vi "http handle content data.vi"(6 "exec queue":refnum<queue>, 9 "server properties":T1={"max url size"=8000, "max header"=8000, "timeout ms"=5000, "max data size"=104857600}, 10 "application request":T2, 11 "TCP Network Connection in":refnum<k5>) -> (3 "abort":bool)   [LabVIEW 2016, in "Basic HTTP server.lvclass"]
uses:
  Basic HTTP server.lvclass
  http request.ctl
  http method.ctl
  HTTP headers/http header data.ctl
  http server properties.ctl
  http chunked encoding state.ctl
  <vilib>/dlg_ctls.llb/Space Constant.vi
  HTTP headers/http add header to set.vi
  HTTP headers/http headers.lvlib
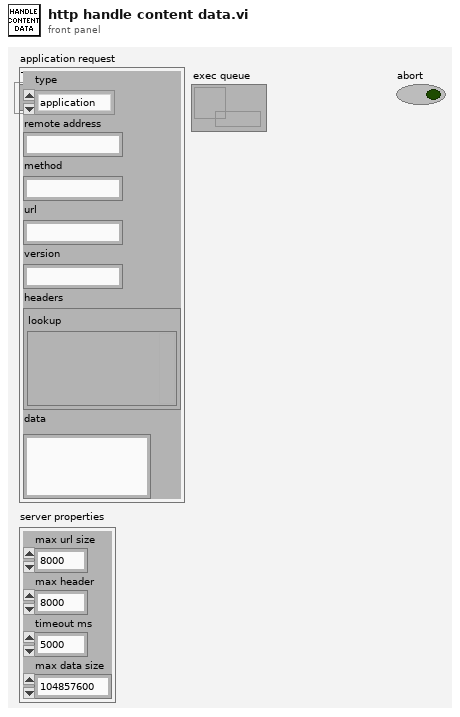
[diagram p1: front panel]
types:
  T1 = typedef "Basic HTTP server.lvclass/http server properties.ctl" = cluster{"max url size":i32, "max header":i32, "timeout ms":i32, "max data size":i32}
  T2 = typedef "Basic HTTP server.lvclass/http request.ctl" = cluster{"type":T3, "remote address":string, "method":string, "url":string, "version":string, "headers":T4, "data":string}
  T3 = typedef "Basic HTTP server.lvclass/http method.ctl" = enum16{"application", "error", "upgrade", "expect"}
  T4 = typedef "http headers.lvlib/http header data.ctl" = cluster{"lookup":variant}
  T5 = typedef "Basic HTTP server.lvclass/http chunked encoding state.ctl" = enum16{"length", "data", "trailer"}
  T6 = enum16{"Standard", "Buffered", "CRLF", "Immediate"}
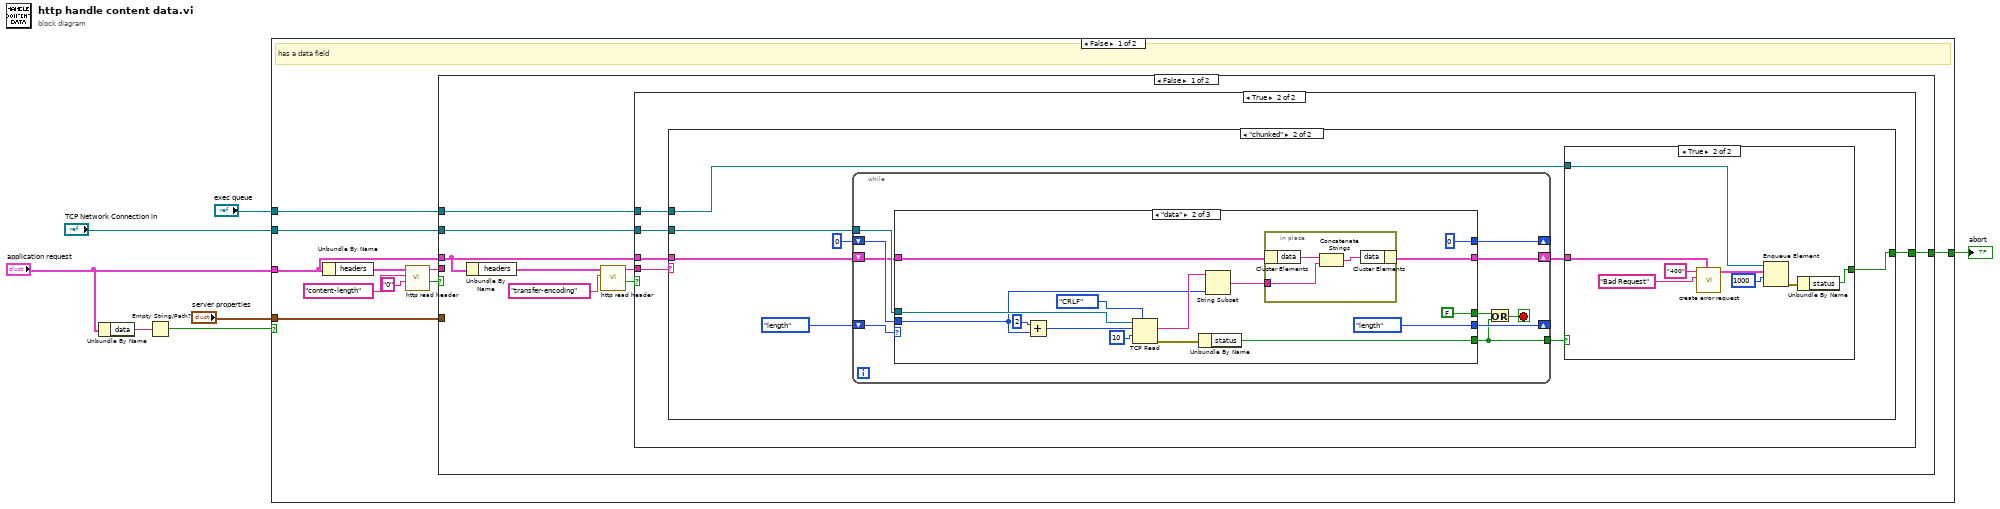
[diagram p0: block diagram]
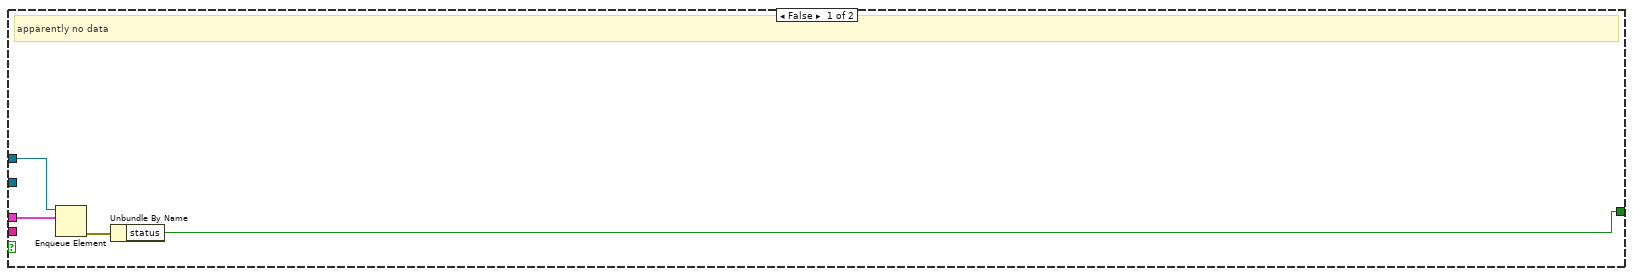
[diagram p2: hidden frame]
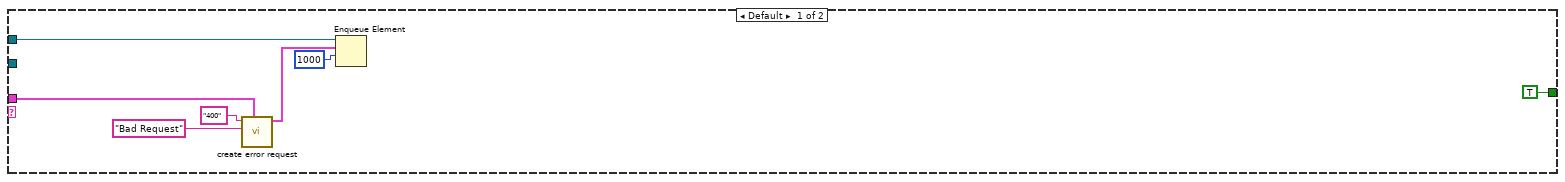
[diagram p3: hidden frame]
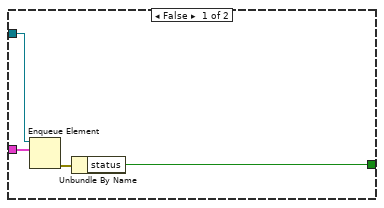
[diagram p4: hidden frame]
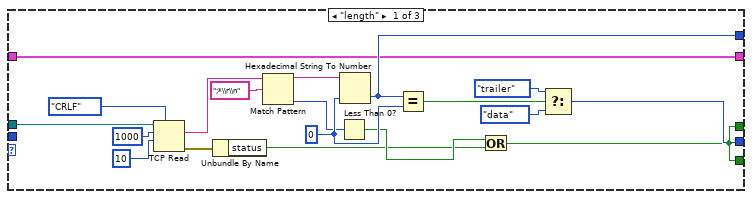
[diagram p5: hidden frame]
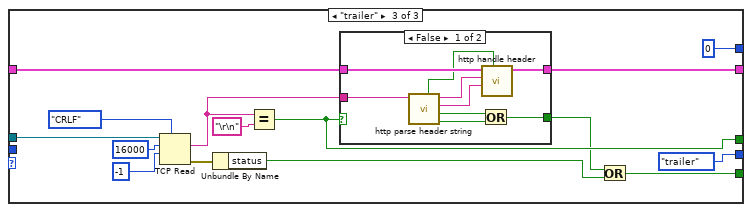
[diagram p6: hidden frame]
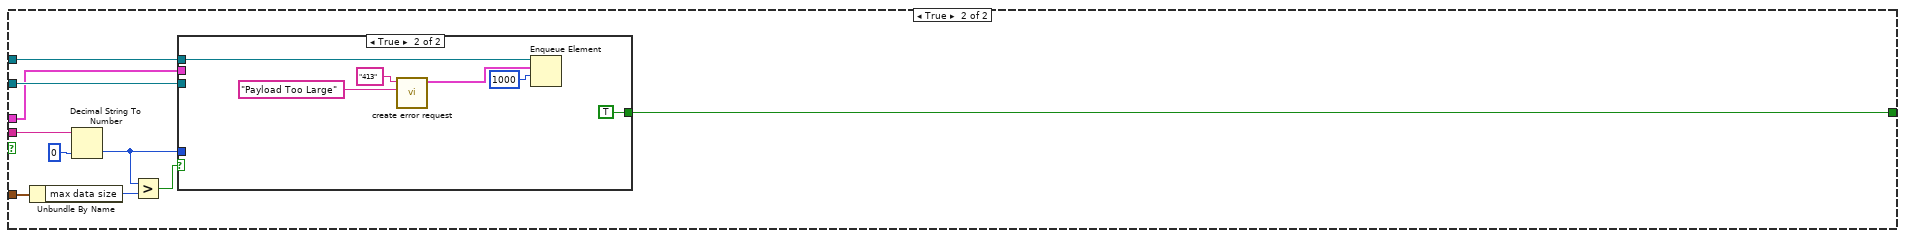
[diagram p8: hidden frame]
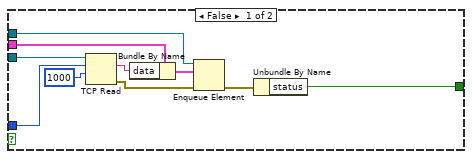
[diagram p9: hidden frame]
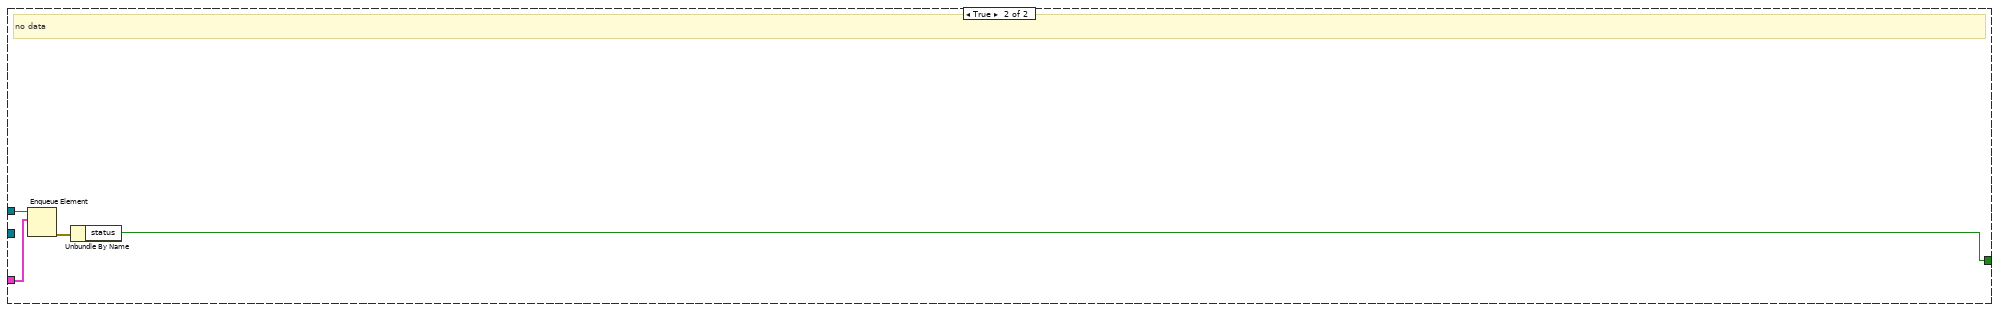
[diagram p10: hidden frame]
diagram:
  n1 = Unbundle By Name("application request") -> ("data"=w2:string)
  n2 = Empty String/Path?(string/path=w2) -> (empty?=w1:bool)
  n3 = case shown="False" w1 {
    tunnel: "TCP Network Connection in" -> [w17 _]
    tunnel: [w16 w160] -> w6
    tunnel: "server properties" -> [w15 _]
    tunnel: "exec queue" -> [w14 w162]
    tunnel: "application request" -> [w13 w163]
    frame False {
      # "has a data field"
      n4 = Unbundle By Name(w13) -> ("headers"=w12:T4)
      n5 = call "http read header.vi"("default value"="0", "header field name"="content-length" ("name"), "headers"=w12) -> ("found"=w10:bool, "value"=w9:string)  [unwired: 7 in]
      n6 = case shown="False" w10 {
        tunnel: w13 -> [w24 w135]
        tunnel: w17 -> [w23 w142]
        tunnel: [w25 w141] -> w16
        tunnel: w15 -> [_ w140]
        tunnel: w14 -> [w22 w136]
        tunnel: w9 -> [_ w134]
        frame False {
          n7 = Unbundle By Name(w24) -> ("headers"=w21:T4)
          n8 = call "http read header.vi"("header field name"="transfer-encoding" ("name"), "headers"=w21) -> ("found"=w19:bool, "value"=w18:string)  [unwired: 8 in]
          n9 = case shown="True" w19 {
            tunnel: [w26 w34] -> w25
            tunnel: w24 -> [w29 w31]
            tunnel: w23 -> [_ w33]
            tunnel: w22 -> [w28 w32]
            tunnel: w18 -> [_ w30]
            frame False {
              # "apparently no data"
              n10 = Enqueue Element(queue=w28, element=w29) -> (error out=w27:errorcluster)  [unwired: 2 in, 2 out]
              n11 = Unbundle By Name(w27) -> ("status"=w26:bool)
            }
            frame True {
              n12 = case shown="\"chunked\"" w30 {
                tunnel: [TRUE w42] -> w34
                tunnel: w31 -> [w35 w46]
                tunnel: w33 -> [_ w48]
                tunnel: w32 -> [w36 w43]
                frame Default {
                  n13 = call "create error request.vi"("incoming request"=w35, "reason"="Bad Request" ("status string"), "code"="400") -> ("element"=w38:T2)  [unwired: 8 in]
                  n14 = Enqueue Element(queue=w36, element=w38, timeout in ms (-1)=1000) -> ()  [unwired: 1 in, 3 out]
                }
                frame "chunked" {
                  n15 = while {
                    shift-right: [w69] -> _
                    shift-left: http_chunked_encoding_state."length" -> [w71]
                    tunnel: w48 -> [w70]
                    shift-right: [w67] -> _
                    shift-left: 0 ("default (0 I32)") -> [w66]
                    shift-right: [w64] -> w44
                    shift-left: w46 -> [w65]
                    tunnel: [w62] -> w45
                    stop <- w63 stop-if-true
                    n16 = case shown="\"data\"" w71 {
                      tunnel: w70 -> [w90 w103 w120]
                      tunnel: [w77 http_chunked_encoding_state."length" http_chunked_encoding_state."trailer"] -> w69
                      tunnel: [w73 FALSE w114] -> w68
                      tunnel: [w82 0 0] -> w67
                      tunnel: w66 -> [_ w99 _]
                      tunnel: w65 -> [w76 w92 w112]
                      tunnel: [w76 w91 w113] -> w64
                      tunnel: [w73 w93 w111] -> w62
                      frame "length" {
                        w83 = 0 ("default (0 I32)")
                        n17 = TCP Read(connection ID=w90, bytes to read=1000, 7:T6."CRLF" ("mode (standard)"), 9:10 ("timeout ms (25000)")) -> (data out=w86:string, error out=w74:errorcluster)  [unwired: 1 in, 1 out]
                        n18 = Unbundle By Name(w74) -> ("status"=w72:bool)
                        n19 = Match Pattern(string=w86, regular expression=";*\\r\\n") -> (before substring=w84:string, offset past match=w81:i32)  [unwired: 1 in, 2 out]
                        n20 = Less Than 0?(x=w81) -> (x < 0?=w75:bool)
                        n21 = Hexadecimal String To Number(string=w84, default (0uL)=w83) -> (number=w82:i32)  [unwired: 1 in, 1 out]
                        n22 = Equal?(x=w82, y=w83) -> (x = y?=w80:bool)
                        n23 = Or(x=w75, y=w72) -> (x .or. y?=w73:bool)
                        n24 = Select(t=http_chunked_encoding_state."trailer", s=w80, f=http_chunked_encoding_state."data") -> (s? t:f=w77:T5)
                      }
                      frame "data" {
                        n25 = Add(x=2, y=w99) -> (x+y=w102:i32)
                        n26 = TCP Read(connection ID=w103, bytes to read=w102, 7:T6."CRLF" ("mode (standard)"), 9:10 ("timeout ms (25000)")) -> (data out=w100:string, error out=w94:errorcluster)  [unwired: 1 in, 1 out]
                        n27 = Unbundle By Name(w94) -> ("status"=w93:bool)
                        n28 = String Subset(string=w100, length (rest)=w99) -> (substring=w98:string)  [unwired: 1 in]
                        n29 = in-place {
                          in-place-border: w98 -> [w108]
                          n30 = in-place-cluster #1(w92) -> ("data"=w107:string)
                          n31 = Concatenate Strings(w107, w108) -> (w106:string)
                          n32 = in-place-cluster #1("data"=w106) -> (w91:T2)
                        }
                      }
                      frame "trailer" {
                        n33 = TCP Read(connection ID=w120, bytes to read=16000, 7:T6."CRLF" ("mode (standard)"), 9:-1 ("timeout ms (25000)")) -> (data out=w109:string, error out=w118:errorcluster)  [unwired: 1 in, 1 out]
                        n34 = Unbundle By Name(w118) -> ("status"=w117:bool)
                        n35 = Equal?(x=w109, y="\r\n" ("x")) -> (x = y?=w114:bool)
                        n36 = case shown="False" w114 {
                          tunnel: [w132 w133] -> w113
                          tunnel: w112 -> [w131 w133]
                          tunnel: [w127 _] -> w110
                          tunnel: w109 -> [w128 _]
                          frame False {
                            n37 = call "http parse header string.vi"("raw string"=w128) -> ("no field name"=w126:bool, "no crlf"=w130:bool, "header field data"=w129:string, "header field name"=w125:string, "continuation"=w124:bool)  [unwired: 6 in]
                            n38 = Or(x=w130, y=w126) -> (x .or. y?=w127:bool)
                            n39 = call "http handle header.vi"("continuation"=w124, "header field data"=w129, "header field name"=w125, "application request in"=w131) -> ("application request out"=w132:T2)  [unwired: 7 in]
                          }
                          frame True {
                          }
                        }
                        n40 = Or(x=w110, y=w117) -> (x .or. y?=w111:bool)
                      }
                    }
                    n41 = Or(x=w68, y=w62) -> (x .or. y?=w63:bool)
                  }
                  n42 = case shown="True" w45 {
                    tunnel: w44 -> [w52 w55]
                    tunnel: w43 -> [w53 w56]
                    tunnel: [w50 w61] -> w42
                    frame False {
                      n43 = Enqueue Element(queue=w53, element=w52) -> (error out=w51:errorcluster)  [unwired: 2 in, 2 out]
                      n44 = Unbundle By Name(w51) -> ("status"=w50:bool)
                    }
                    frame True {
                      n45 = call "create error request.vi"("incoming request"=w55, "reason"="Bad Request" ("status string"), "code"="400") -> ("element"=w59:T2)  [unwired: 8 in]
                      n46 = Enqueue Element(queue=w56, element=w59, timeout in ms (-1)=1000) -> (error out=w54:errorcluster)  [unwired: 1 in, 2 out]
                      n47 = Unbundle By Name(w54) -> ("status"=w61:bool)
                    }
                  }
                }
              }
            }
          }
        }
        frame True {
          n48 = Unbundle By Name(w140) -> ("max data size"=w139:i32)
          n49 = Decimal String To Number(string=w134, default (0L)=0 ("default (0 I32)")) -> (number=w138:i32)  [unwired: 1 in, 1 out]
          n50 = Greater?(x=w138, y=w139) -> (0:w137:bool)
          n51 = case shown="True" w137 {
            tunnel: w142 -> [w153 _]
            tunnel: [w151 TRUE ("status")] -> w141
            tunnel: w135 -> [w150 _]
            tunnel: w138 -> [w147 _]
            tunnel: w136 -> [w145 w156]
            frame False {
              n52 = TCP Read(connection ID=w153, bytes to read=w147, 9:1000 ("timeout ms (25000)")) -> (data out=w149:string, error out=w148:errorcluster)  [unwired: 2 in, 1 out]
              n53 = Bundle By Name(cluster=w150, "data"=w149) -> (w144:T2)
              n54 = Enqueue Element(queue=w145, element=w144, error in (no error)=w148) -> (error out=w146:errorcluster)  [unwired: 1 in, 2 out]
              n55 = Unbundle By Name(w146) -> ("status"=w151:bool)
            }
            frame True {
              n56 = call "create error request.vi"("reason"="Payload Too Large" ("status string"), "code"="413") -> ("element"=w155:T2)  [unwired: 9 in]
              n57 = Enqueue Element(queue=w156, element=w155, timeout in ms (-1)=1000) -> ()  [unwired: 1 in, 3 out]
            }
          }
        }
      }
    }
    frame True {
      # "no data"
      n58 = Enqueue Element(queue=w162, element=w163) -> (error out=w161:errorcluster)  [unwired: 2 in, 2 out]
      n59 = Unbundle By Name(w161) -> ("status"=w160:bool)
    }
  }
  "abort" <- w6
